vi "ARDUINO_LINX_SWAY.vi"() -> ()   [LabVIEW 2016]
uses:
  <vilib>/MakerHub/LINX/Private/Type Defs/Interface.ctl
  <vilib>/MakerHub/LINX/Public/Sensors/Accelerometer/MPU60X0/Clock Source.ctl
  <vilib>/MakerHub/LINX/Private/Type Defs/User Platform.ctl
  <vilib>/MakerHub/LINX/Public/Sensors/Accelerometer/MPU60X0/DeviceAddresses.ctl
  <vilib>/MakerHub/LINX/Public/Sensors/Accelerometer/MPU60X0/AccelFullScaleRanges.ctl
  <vilib>/MakerHub/LINX/Public/Sensors/Accelerometer/MPU60X0/GyroFullScaleRanges.ctl
  <vilib>/MakerHub/LINX/Public/Initialize.vi
  <vilib>/MakerHub/LINX/LMH-LINX.lvlib
  <vilib>/MakerHub/LINX/Public/Sensors/Accelerometer/MPU60X0/MPU60X0.lvlib
  <vilib>/Platform/NI_3dgraph.lvlib
panel:
  out "Waveform kk 2":T1(graph)
  out "Waveform kk":T1(graph)
  out "Path Length":dbl
  out "vector error":errorcluster
  in  "Plot of roll and pitch":refnum<k7>(container)
  out "XY Graph":cluster{"Y":dbl[], "Y":dbl[]}[](graph)
  out "error out":errorcluster
  out "MATLAB Error":errorcluster
  out "Error Out":errorcluster
  in  "?":bool
  in  "I2C Channel":u8
  in  "Clock Source":T2
  in  "Interface":T3
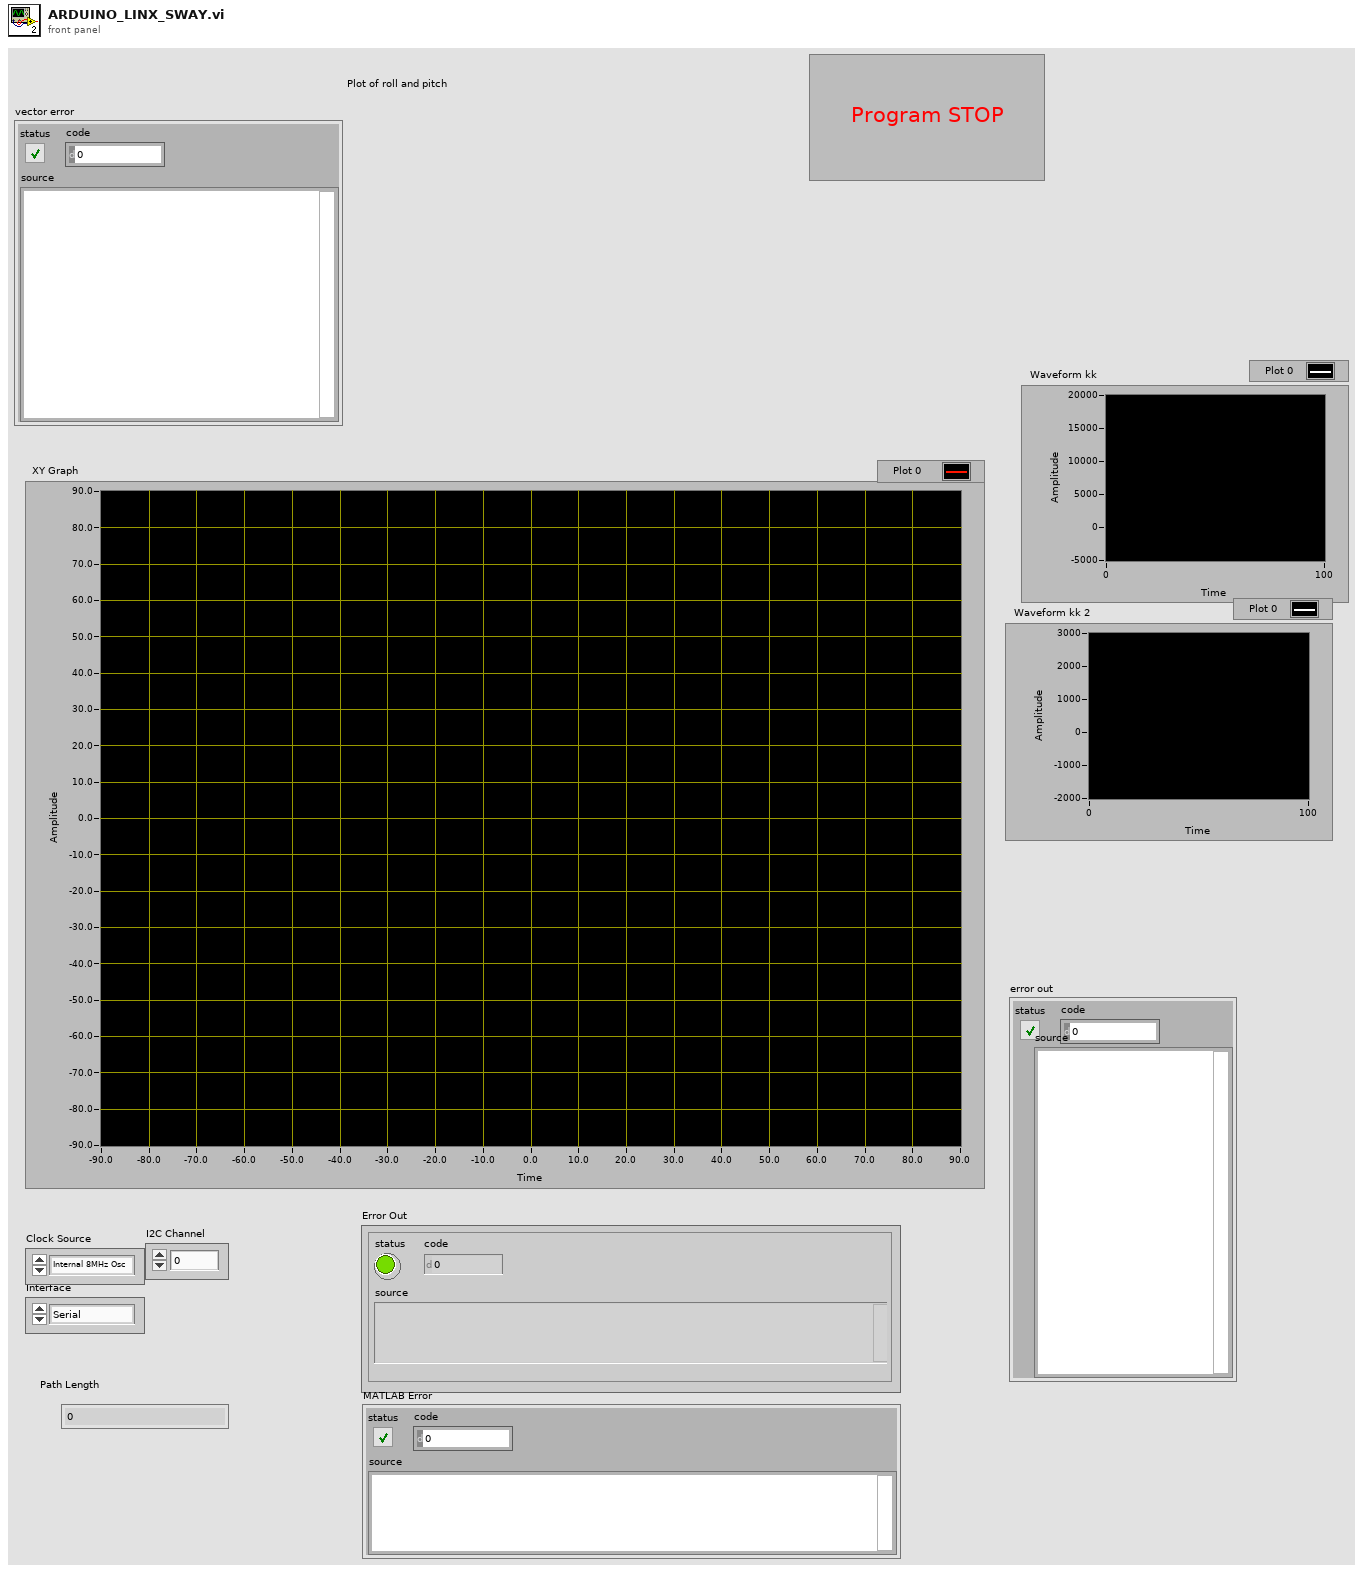
[diagram p1: front panel]
types:
  T1 = cluster{"X Axis":i16, "Y Axis":i16, "Z Axis":i16}
  T2 = typedef "LMH-LINX.lvlib/MPU60X0.lvlib/Clock Source.ctl" = enum8{"Internal 8MHz Osc", "PLL with X Gyro Ref", "PLL with Y Gyro Ref", "PLL with Z Gyro Ref", "PLL with ext 32.768 KHz Ref", "PLL with ext 19.2 MHz Ref", "Reserved", "Hold in reset"}
  T3 = typedef "LMH-LINX.lvlib/Interface.ctl" = enum16{"Serial", "TCP"}
  T4 = typedef "LMH-LINX.lvlib/MPU60X0.lvlib/DeviceAddresses.ctl" = enum16{"0x68", "0x69"}
  T5 = typedef "LMH-LINX.lvlib/MPU60X0.lvlib/GyroFullScaleRanges.ctl" = enum8{"±250 °/s", "±500 °/s", "±1000 °/s", "±2000 °/s"}
  T6 = typedef "LMH-LINX.lvlib/MPU60X0.lvlib/AccelFullScaleRanges.ctl" = enum16{"±2g", "±4g", "±8g", "±16g"}
  T7 = typedef "LMH-LINX.lvlib/User Platform.ctl" = enum16{"Default", "Remote", "Local"}
  T8 = typedef "LMH-LINX.lvlib/LINX Ref.ctl" = cluster{"IO":T9, "Interface":T3, "LINX Device Config":T10}
  T9 = typedef "LMH-LINX.lvlib/Platform.ctl" = enum16{"Remote", "Local"}
  T10 = typedef "LMH-LINX.lvlib/Device.lvlib/LINX Device Config.ctl" = cluster{"Interface":T3, "COM Port":refnum<visa-resource-name>, "TCP Configuration":T11, "Device Family":u8, "Device ID":u8, "Device Name":string, "TCP Ref":refnum<k5>, "Channels":T12}
  T11 = typedef "LMH-LINX.lvlib/Device.lvlib/TCP Config.ctl" = cluster{"IP Address":string, "Port":u16}
  T12 = typedef "LMH-LINX.lvlib/Channels.ctl" = cluster{"DI":u8[], "DO":u8[], "AI":u8[], "AO":u8[], "PWM":u8[], "QE":u8[], "UART":u8[], "I2C 2":u8[], "SPI":u8[], "CAN":u8[], "Servo":u8[], "AI Ref (V)":dbl, "AI Resolution (Bits)":u8, "AO Ref (V)":dbl, "AO Resolution (Bits)":u8}
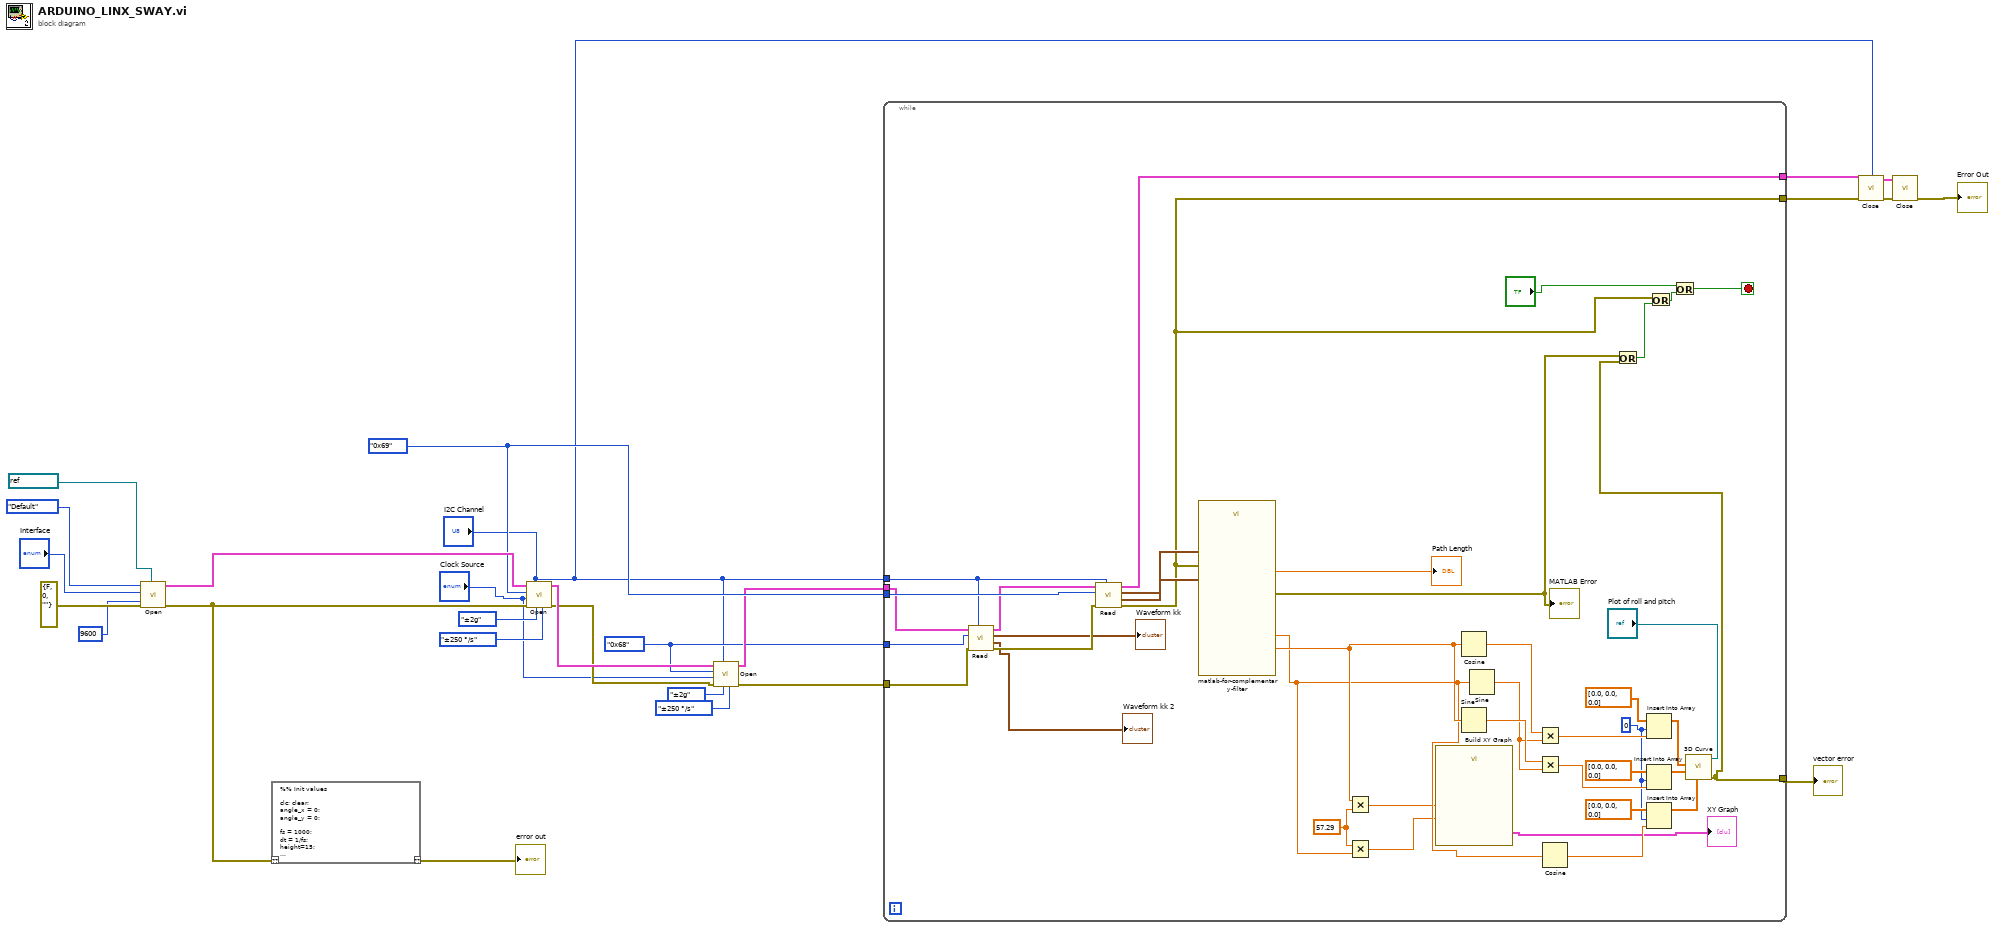
[diagram p0: block diagram]
diagram:
  w2 = DeviceAddresses."0x68" ("I2C Slave Address")
  w20 = DeviceAddresses."0x69" ("Device Address")
  n1 = call-poly <vilib>:"Open.vi"("Baud Rate Override"=u32 9600, "Serial Port"=refnum<visa-resource-name> "COM3", "Error In"=errorcluster {"status"=FALSE, "code"=0, "source"=""}, "Interface"="Interface", "IO"=User_Platform."Default") -> ("Error Out"=w14:errorcluster, "LINX Resource"=w23:T8)  [unwired: 4 in, 1 out]
  n2 = script code="%% Init values\n\nclc; clear;\nangle_x = 0;\nangle_y = 0;\n\nfs = 1000;\ndt = 1/fs;\nheight=15;\n\nx_mag=0; \ny_mag=0; \n\np_length = 0;\n\ncalc=0;"("??"=w14) -> ("??"=→"error out":errorcluster)
  n3 = call <vilib>:"Open.vi"("Gyro Full Scale Range"=GyroFullScaleRanges."±250 °/s", "Accel Full Scale Range"=AccelFullScaleRanges."±2g", "I2C Channel"="I2C Channel", "Error In"=w14, "Clock Source"="Clock Source", "I2C Slave Address"=w20, "LINX Resource"=w23) -> ("Error Out"=w5:errorcluster, "LINX Resource"=w9:T8)  [unwired: 3 in]
  n4 = call <vilib>:"Open.vi"("Gyro Full Scale Range"=GyroFullScaleRanges."±250 °/s", "Accel Full Scale Range"=AccelFullScaleRanges."±2g", "I2C Channel"="I2C Channel", "Error In"=w5, "Clock Source"="Clock Source", "I2C Slave Address"=w2, "LINX Resource"=w9) -> ("Error Out"=w4:errorcluster, "LINX Resource"=w8:T8)  [unwired: 3 in]
  n5 = while {
    tunnel: w8 -> [w34]
    tunnel: w20 -> [w66]
    tunnel: [w65] -> w19
    tunnel: [w41] -> w17
    tunnel: [w42] -> w10
    tunnel: w4 -> [w31]
    tunnel: w2 -> [w32]
    tunnel: "I2C Channel" -> [w27]
    stop <- w45 stop-if-true
    w49 = 57.29 ("y")
    w51 = 0 ("index")
    n6 = call <vilib>:"Read.vi"("I2C Channel"=w27, "Error In"=w31, "I2C Slave Address"=w32, "LINX Resource"=w34) -> ("Error Out"=w30:errorcluster, "Gyro  Data (dps)"=→"Waveform kk 2":T1, "Acceleration Data (g)"=→"Waveform kk":T1, "LINX Resource"=w33:T8)  [unwired: 3 in, 1 out]
    n7 = call <vilib>:"Read.vi"("I2C Channel"=w27, "Error In"=w30, "I2C Slave Address"=w66, "LINX Resource"=w33) -> ("Error Out"=w41:errorcluster, "Gyro  Data (dps)"=w63:T1, "Acceleration Data (g)"=w64:T1, "LINX Resource"=w65:T8)  [unwired: 3 in, 1 out]
    n8 = call "matlab-for-complementary-filter.vi"("Acceleration Data (g)"=w64, "Gyro  Data (dps)"=w63, "error in (no error)"=w41) -> ("angle_y"=w50:dbl, "Path Length"=→"Path Length":dbl, "angle_x"=w48:dbl, "error out"=w43:errorcluster)  [unwired: 11 in, 2 out]
    "MATLAB Error" <- w43
    n9 = Multiply(x=w50, y=w49) -> (x*y=w37:dbl)
    n10 = Multiply(x=w49, y=w48) -> (x*y=w36:dbl)
    n11 = call "Build XY Graph"("Y Input"=w36, "X Input"=w37) -> ("XY Graph"=→"XY Graph":cluster{"X":dbl[], "Y":dbl[]}[])  [unwired: 8 in, 1 out]
    n12 = Cosine(x=w50) -> (cos(x)=w62:dbl)
    n13 = Sine(x=w50) -> (sin(x)=w57:dbl)
    n14 = Sine(x=w48) -> (sin(x)=w56:dbl)
    n15 = Multiply(x=w62, y=w56) -> (x*y=w59:dbl)
    n16 = Multiply(x=w57, y=w56) -> (x*y=w55:dbl)
    n17 = Cosine(x=w48) -> (cos(x)=w53:dbl)
    n18 = Insert Into Array(array=dbl[] [0.0, 0.0, 0.0], index=w51, new element=w59) -> (w47:dbl[])
    n19 = Insert Into Array(array=dbl[] [0.0, 0.0, 0.0], index=w51, new element=w55) -> (w46:dbl[])
    n20 = Insert Into Array(array=dbl[] [0.0, 0.0, 0.0], index=w51, new element=w53) -> (w52:dbl[])
    n21 = call <vilib>:"3D Curve.vi"("z vector"=w52, "y vector"=w46, "x vector"=w47, "3D graph"="Plot of roll and pitch") -> ("error out"=w42:errorcluster)  [unwired: 6 in, 1 out]
    n22 = Or(x=w43, y=w42) -> (x .or. y?=w44:bool)
    n23 = Or(x=w41, y=w44) -> (x .or. y?=w39:bool)
    n24 = Or(x="?", y=w39) -> (x .or. y?=w45:bool)
  }
  "vector error" <- w10
  n25 = call <vilib>:"Close.vi"("I2C Channel (0)"="I2C Channel", "Error In"=w17, "LINX Resource"=w19) -> ("Error Out"=w16:errorcluster, "LINX Resource"=w18:T8)  [unwired: 7 in]
  n26 = call <vilib>:"Close.vi"("Error In"=w16, "LINX Resource"=w18) -> ("Error Out"=→"Error Out":errorcluster)  [unwired: 9 in]
